vi "element_editor_validate_specs.vi"(9 "Vali File Loaded?":refnum<vi>, 10 "Parameters Tree":refnum<vi>) -> (0 "validationErrors":string, 1 "Valid?":bool, 3 "validationMsg":string)   [LabVIEW 2019]
uses:
  lib/libSpecValiReader/libSpecValiReader.lvlib
panel:
  out "Specifications":string
  # "*******************************************************************\nBiogas Plant Control\n\nAuthor: Paul Zügel\nGCSC-Frankfurt am Main 2020\n\n*******************************************************************"
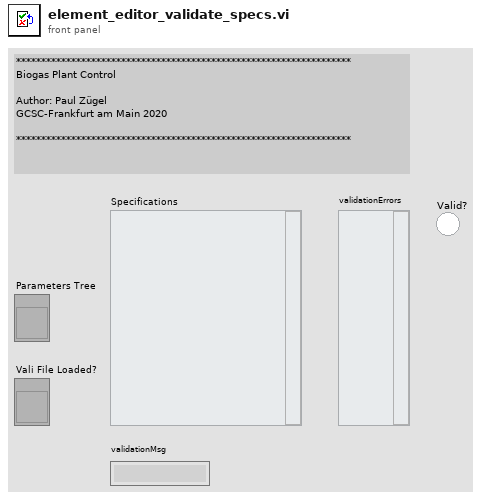
[diagram p1: front panel]
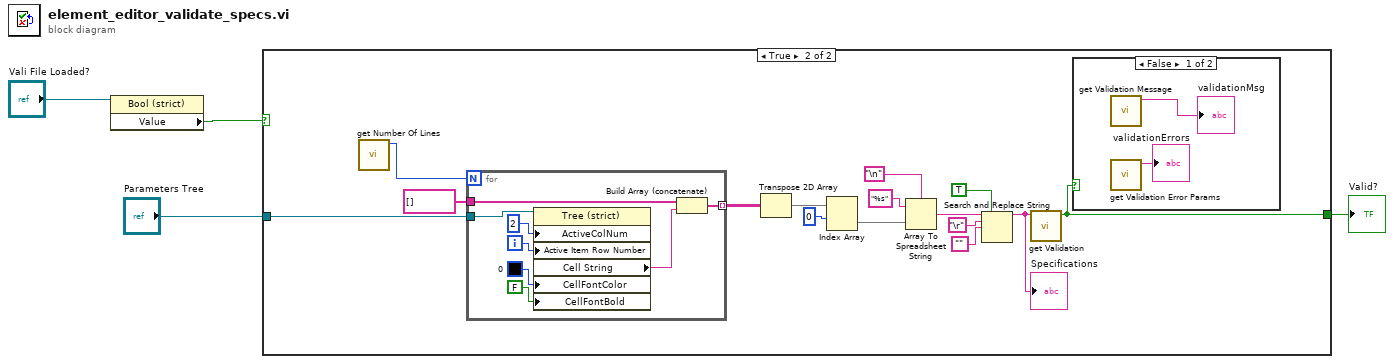
[diagram p0: block diagram]
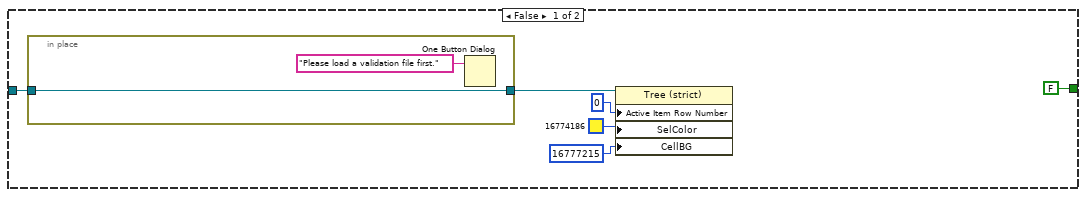
[diagram p2: hidden frame]
diagram:
  n1 = property class="Bool (strict)"(reference="Vali File Loaded?") -> ("Value"=w1:bool)  [unwired: 1 in, 2 out]
  n2 = case shown="True" w1 {
    tunnel: "Parameters Tree" -> [w6 w20]
    tunnel: [FALSE w19] -> w3
    frame False {
      n3 = in-place {
        in-place-border: w6 -> [w11]
        in-place-border: [w11] -> w5
        n4 = One Button Dialog(message="Please load a validation file first.") -> ()  [unwired: 1 in, 1 out]
      }
      n5 = property on="Property Node" class="Tree (strict)"(reference=w5, "Active Item Row Number"=0 ("Active Item:Row Number"), "SelColor"=u32 16774186, "CellBG"=u32 16777215 ("Active Cell:Background Color")) -> ()  [unwired: 1 in, 2 out]
    }
    frame True {
      n6 = call "get Number Of Lines.vi"() -> ("function return"=w13:i32)  [unwired: 10 in, 1 out]
      n7 = for {
        N: w13 -> [_]
        tunnel: string[] [] ("Empty Val Arr") -> [w33]
        tunnel: [w32] -> w26 mode=indexing
        tunnel: w20 -> [w30]
        i -> [w35]
        n8 = property on="Property Node" class="Tree (strict)"(reference=w30, "ActiveColNum"=2 ("Active Cell:Active Column Number"), "Active Item Row Number"=w35, "CellFontColor"=u32 0 ("Active Cell:Cell Font:Color"), "CellFontBold"=FALSE ("Active Cell:Cell Font:Bold")) -> ("Cell String"=w31:string)  [unwired: 1 in, 2 out]
        n9 = Build Array (concatenate)(w33, w31) -> (w32:string[])
      }
      n10 = Transpose 2D Array(2D array=w26) -> (transposed array=w25:string[][])
      n11 = Index Array(array=w25, index (row)=0) -> (element=w24:string[])  [unwired: 1 in]
      n12 = Array To Spreadsheet String(delimiter (Tab)="\n", array=w24, 3:"%s" ("format string")) -> (spreadsheet string=w18:string)
      n13 = Search and Replace String(replace all?=TRUE ("replace all? (F)"), input string=w18, search string="\r", replace string="") -> (result string=w17:string)  [unwired: 4 in, 3 out]
      "Specifications" <- w17
      n14 = call "get Validation.vi"("specs"=w17) -> ("function return"=w19:bool)  [unwired: 9 in, 1 out]
      n15 = case shown="False" w19 {
        frame False {
          n16 = call "get Validation Message.vi"() -> ("function return"=→"validationMsg":string)  [unwired: 10 in, 1 out]
          n17 = call "get Validation Error Params.vi"() -> ("function return"=→"validationErrors":string)  [unwired: 10 in, 1 out]
        }
        frame True {
        }
      }
    }
  }
  "Valid?" <- w3
